vi "MakeConsoleErrorCluster.vi"(6 "Error Cluster in":T3, 8 "TabControl in":refnum<vi>, 9 "# of Errors":i32, 10 "Log":T2={"Sent"="", "Reply"="", "MethodName"="", "success"=FALSE, "XML Direction 1"="", "XML Direction 2"="", "VI Name"="", "close reference"={"status"=FALSE, "code"=0, "source"=""}, "release queue"={"status"=FALSE, "code"=0, "source"=""}, "release notification"={"status"=FALSE, "code"=0, "source"=""}, "varaiant to data"={"status"=FALSE, "code"=0, "source"=""}, "console error"={"status"=FALSE, "code"=0, "source"=""}, "Time Stamp"="", "ROS"={"topic port"=0, "Node"="", "topic"="", "type"="", "node port"=0, "error "={"status"=FALSE, "code"=0, "source"=""}, "Direction"=enum."Node", "Update (ms)"=1, "write queue"=1}}, 11 "Number Cluster in":T4) -> (1 "Console Errors":T5(array[cluster]), 2 "Error Cluster Out":T3, 3 "Number Cluster out":T4)   [LabVIEW 2012]
uses:
  <userlib>/ROSforLV/ROS/Code/SubVIs/_ROSDirection.ctl
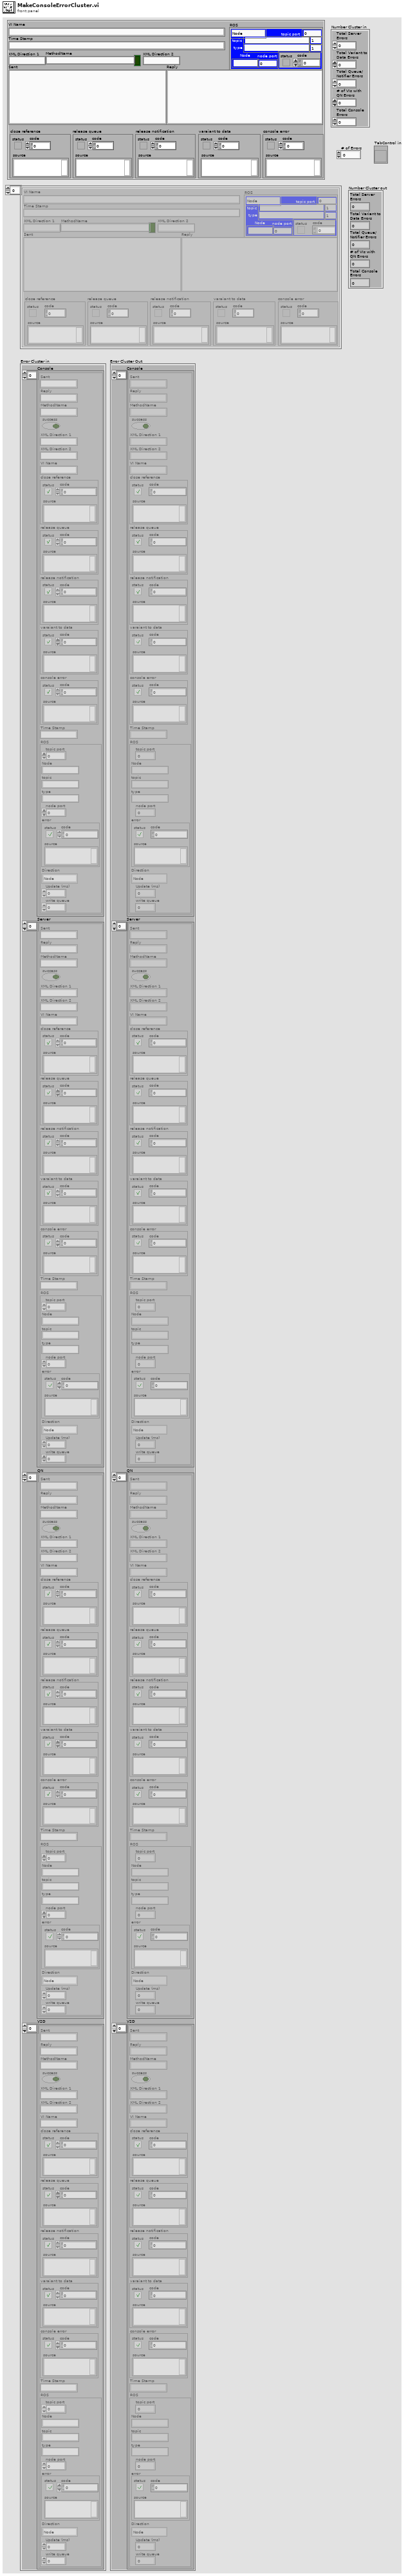
[diagram p1: front panel]
types:
  T1 = typedef "_ROSDirection.ctl" = enum16{"Node", "Publisher", "Subscriber", "Service Client"}
  T2 = cluster{"Sent":string, "Reply":string, "MethodName":string, "success":bool, "XML Direction 1":string, "XML Direction 2":string, "VI Name":string, "close reference":errorcluster, "release queue":errorcluster, "release notification":errorcluster, "varaiant to data":errorcluster, "console error":errorcluster, "Time Stamp":string, "ROS":cluster{"topic port":u16, "Node":string, "topic":string, "type":string, "node port":u32, "error ":errorcluster, "Direction":T1, "Update (ms)":u16, "write queue":u16}}
  T3 = cluster{"Console":cluster{"Sent":string, "Reply":string, "MethodName":string, "success":bool, "XML Direction 1":string, "XML Direction 2":string, "VI Name":string, "close reference":errorcluster, "release queue":errorcluster, "release notification":errorcluster, "varaiant to data":errorcluster, "console error":errorcluster, "Time Stamp":string, "ROS":cluster{"topic port":u16, "Node":string, "topic":string, "type":string, "node port":u32, "error ":errorcluster, "Direction":T1, "Update (ms)":u16, "write queue":u16}}[], "Server":cluster{"Sent":string, "Reply":string, "MethodName":string, "success":bool, "XML Direction 1":string, "XML Direction 2":string, "VI Name":string, "close reference":errorcluster, "release queue":errorcluster, "release notification":errorcluster, "varaiant to data":errorcluster, "console error":errorcluster, "Time Stamp":string, "ROS":cluster{"topic port":u16, "Node":string, "topic":string, "type":string, "node port":u32, "error ":errorcluster, "Direction":T1, "Update (ms)":u16, "write queue":u16}}[], "QN":cluster{"Sent":string, "Reply":string, "MethodName":string, "success":bool, "XML Direction 1":string, "XML Direction 2":string, "VI Name":string, "close reference":errorcluster, "release queue":errorcluster, "release notification":errorcluster, "varaiant to data":errorcluster, "console error":errorcluster, "Time Stamp":string, "ROS":cluster{"topic port":u16, "Node":string, "topic":string, "type":string, "node port":u32, "error ":errorcluster, "Direction":T1, "Update (ms)":u16, "write queue":u16}}[], "V2D":cluster{"Sent":string, "Reply":string, "MethodName":string, "success":bool, "XML Direction 1":string, "XML Direction 2":string, "VI Name":string, "close reference":errorcluster, "release queue":errorcluster, "release notification":errorcluster, "varaiant to data":errorcluster, "console error":errorcluster, "Time Stamp":string, "ROS":cluster{"topic port":u16, "Node":string, "topic":string, "type":string, "node port":u32, "error ":errorcluster, "Direction":T1, "Update (ms)":u16, "write queue":u16}}[]}
  T4 = cluster{"Total Server\nErrors":i32, "Total Variant to\nData Errors":i32, "Total Queue/\nNotifier Errors":i32, "# of VIs with\nQN Errors":i32, "Total Console\nErrors":i32}
  T5 = cluster{"Sent":string, "Reply":string, "MethodName":string, "success":bool, "XML Direction 1":string, "XML Direction 2":string, "VI Name":string, "close reference":errorcluster, "release queue":errorcluster, "release notification":errorcluster, "varaiant to data":errorcluster, "console error":errorcluster, "Time Stamp":string, "ROS":cluster{"topic port":u16, "Node":string, "topic":string, "type":string, "node port":u32, "error ":errorcluster, "Direction":T1, "Update (ms)":u16, "write queue":u16}}[]
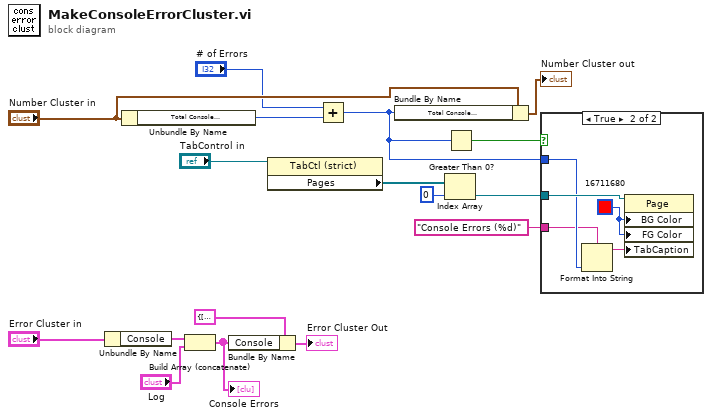
[diagram p0: block diagram]
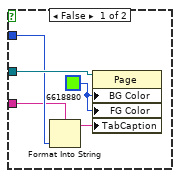
[diagram p2: hidden frame]
diagram:
  n1 = Unbundle By Name("Error Cluster in") -> ("Console"=w11:T5)
  n2 = Unbundle By Name("Number Cluster in") -> ("Total Console\nErrors"=w16:i32)
  n3 = Build Array (concatenate)(w11, "Log") -> (w12:T5)
  "Console Errors" <- w12
  n4 = Bundle By Name(cluster=T3 {"Console"=[], "Server"=[], "QN"=[], "V2D"=[]}, "Console"=w12) -> (→"Error Cluster Out":T3)
  n5 = property on="Property Node" class="TabCtl (strict)"(reference="TabControl in") -> ("Pages"=w6:refnum<vi>[])  [unwired: 1 in, 2 out]
  n6 = Add(x="# of Errors", y=w16) -> (x+y=w1:i32)
  n7 = Bundle By Name(cluster="Number Cluster in", "Total Console\nErrors"=w1) -> (→"Number Cluster out":T4)
  n8 = Index Array(array=w6, index=0) -> (element=w5:refnum<vi>)
  n9 = Greater Than 0?(x=w1) -> (x > 0?=w8:bool)
  n10 = case shown="True" w8 {
    tunnel: w5 -> [w20 w27]
    tunnel: w1 -> [w19 w24]
    tunnel: "Console Errors (%d)" ("format string") -> [w18 w23]
    frame False {
      w22 = u32 6618880
      n11 = Format Into String(format string=w18, w19) -> (resulting string=w21:string)  [unwired: 2 in, 1 out]
      n12 = property on="Property Node" class="Page"(reference=w20, "BG Color"=w22, "FG Color"=w22, "TabCaption"=w21) -> ()  [unwired: 1 in, 2 out]
    }
    frame True {
      w26 = u32 16711680
      n13 = Format Into String(format string=w23, w24) -> (resulting string=w25:string)  [unwired: 2 in, 1 out]
      n14 = property on="Property Node" class="Page"(reference=w27, "BG Color"=w26, "FG Color"=w26, "TabCaption"=w25) -> ()  [unwired: 1 in, 2 out]
    }
  }
